vi "Move Absolute Motor.vi"(6 "Position":dbl min=-2000000000.0 max=2000000000.0 format="%.6f", 7 "timeout":dbl, 8 "error in (no error)":errorcluster, 9 "Axis":i32=1 min=1 max=3, 10 "VISA resource name in":refnum<visa-resource-name>, 11 "ESP302 in":refnum<class "ESP302.lvclass">) -> (0 "error out":errorcluster, 2 "VISA resource name out":refnum<visa-resource-name>, 3 "ESP302 out":refnum<class "ESP302.lvclass">)   [LabVIEW 2020, in "ESP302.lvclass"]
uses:
  ESP302.lvclass
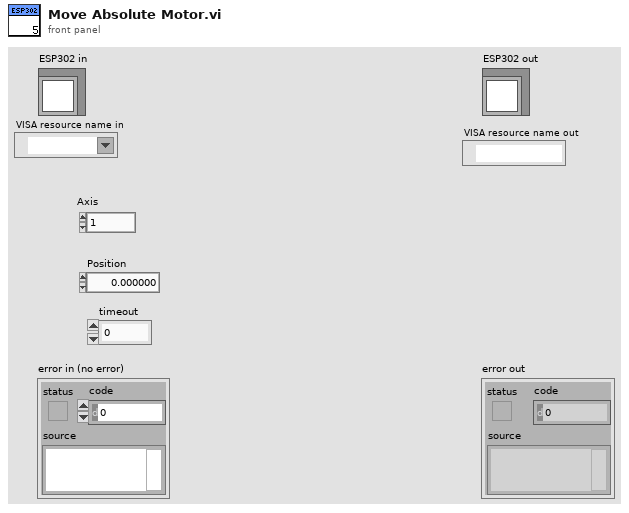
[diagram p1: front panel]
types:
  T1 = typedef "ESP301.lvclass/SettingsTypdef.ctl" = cluster{"devport":string, "Position":cluster{"Axis 1":cluster{"Value":dbl, "Min":dbl, "Max":dbl, "StepSize":dbl, "Tolerance":dbl, "ValueActual":dbl}, "Axis 2":cluster{"Value":dbl, "Min":dbl, "Max":dbl, "StepSize":dbl, "Tolerance":dbl, "ValueActual":dbl}, "Axis 3":cluster{"Value":dbl, "Min":dbl, "Max":dbl, "StepSize":dbl, "Tolerance":dbl, "ValueActual":dbl}}, "Power":cluster{"Axis 1":T2, "Axis 2":T2, "Axis 3":T2}, "Status":cluster{"Axis 1":T3, "Axis 2":T3, "Axis 3":T3}, "Backlash":cluster{"Axis 1":cluster{"Value":dbl, "Min":dbl, "Max":dbl, "StepSize":dbl, "Tolerance":dbl, "ValueActual":dbl}, "Axis 2":cluster{"Value":dbl, "Min":dbl, "Max":dbl, "StepSize":dbl, "Tolerance":dbl, "ValueActual":dbl}, "Axis 3":cluster{"Value":dbl, "Min":dbl, "Max":dbl, "StepSize":dbl, "Tolerance":dbl, "ValueActual":dbl}}, "Home":cluster{"Axis 1":cluster{"Value":dbl, "Min":dbl, "Max":dbl, "StepSize":dbl, "Tolerance":dbl, "ValueActual":dbl}, "Axis 2":cluster{"Value":dbl, "Min":dbl, "Max":dbl, "StepSize":dbl, "Tolerance":dbl, "ValueActual":dbl}, "Axis 3":cluster{"Value":dbl, "Min":dbl, "Max":dbl, "StepSize":dbl, "Tolerance":dbl, "ValueActual":dbl}}, "MoveToHardLimit":cluster{"Axis 1":T4, "Axis 2":T4, "Axis 3":T4}, "relativeMove":cluster{"Axis 1neg":T2, "Axis 2neg":T2, "Axis 3neg":T2, "Axis 1pos":T2, "Axis 2pos":T2, "Axis 3pos":T2}, "stepsize":cluster{"Value":dbl, "Min":dbl, "Max":dbl, "StepSize":dbl, "Tolerance":dbl, "ValueActual":dbl}, "automotoroff":T2, "ResetBeforeMove":T2, "Enable":cluster{"Axis 1":T2, "Axis 2":T2, "Axis 3":T2}, "InitWithDBValues":T2}
  T2 = typedef "OnOffTypeDef.ctl" = enum16{"off", "on"}
  T3 = typedef "status_TypDef.ctl" = enum16{"Not referenced", "Homing", "Moving", "Ready"}
  T4 = typedef "Hardware limit.ctl" = enum16{"pos", "neg"}
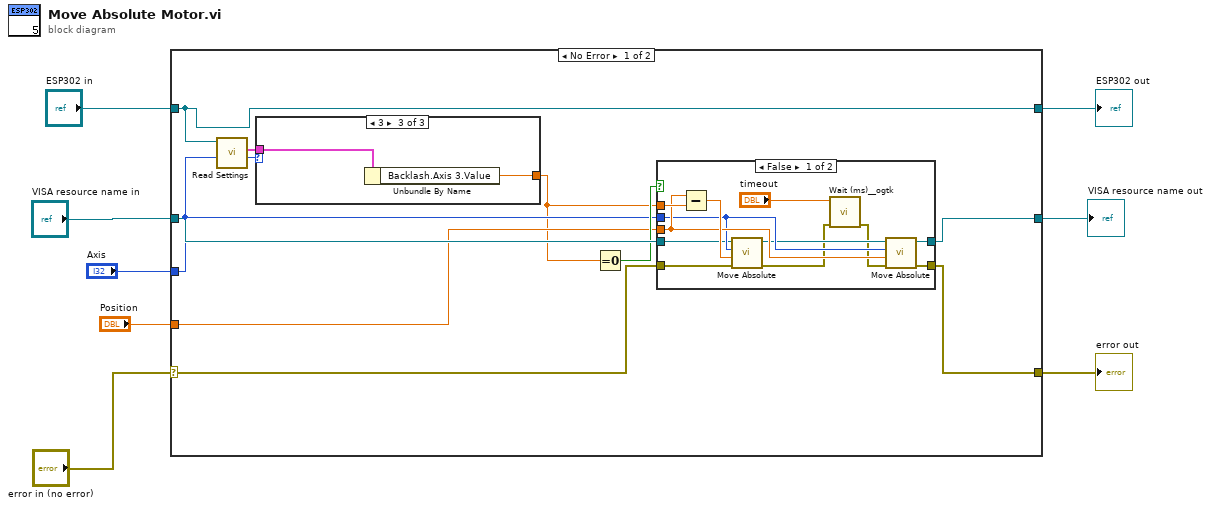
[diagram p0: block diagram]
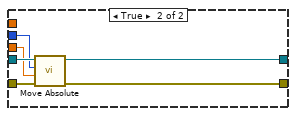
[diagram p2: hidden frame]
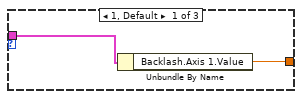
[diagram p3: hidden frame]
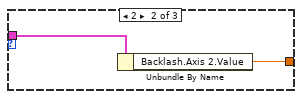
[diagram p4: hidden frame]
diagram:
  n1 = case shown="No Error" "error in (no error)" {
    selector: "error in (no error)" -> [w13 w45]
    tunnel: [w12 w45] -> w7
    tunnel: [w11 w44] -> w5
    tunnel: "ESP302 in" -> [w11 w44]
    tunnel: "VISA resource name in" -> [w18 w43]
    tunnel: [w17 w43] -> w3
    tunnel: "Axis" -> [w15 _]
    tunnel: "Position" -> [w14 _]
    frame No Error {
      n2 = call-dynamic "Read Settings.vi"("ESP301 in"=w11) -> ("Settings"=w10:T1)  [unwired: 8 in, 2 out]
      n3 = case shown="3" w15 {
        tunnel: w10 -> [w37 w40 w42]
        tunnel: [w38 w39 w41] -> w9
        frame 1, Default {
          n4 = Unbundle By Name(w37) -> ("Backlash.Axis 1.Value"=w38:dbl)
        }
        frame 2 {
          n5 = Unbundle By Name(w40) -> ("Backlash.Axis 2.Value"=w39:dbl)
        }
        frame 3 {
          n6 = Unbundle By Name(w42) -> ("Backlash.Axis 3.Value"=w41:dbl)
        }
      }
      n7 = Equal To 0?(x=w9) -> (x = 0?=w16:bool)
      n8 = case shown="False" w16 {
        tunnel: w18 -> [w24 w36]
        tunnel: [w23 w35] -> w17
        tunnel: w15 -> [w26 w34]
        tunnel: w14 -> [w27 w33]
        tunnel: w13 -> [w28 w32]
        tunnel: [w22 w31] -> w12
        tunnel: w9 -> [w30 _]
        frame False {
          n9 = Subtract(x=w27, y=w30) -> (x-y=w29:dbl)
          n10 = call "Move Absolute.vi"("error in (no error)"=w28, "Position (0 units)"=w29, "Axis (1)"=w26, "VISA resource name"=w24) -> ("error out"=w21:errorcluster, "VISA resource name out"=w25:refnum<visa-resource-name>)  [unwired: 2 in]
          n11 = call <userlib>:"Wait (ms)__ogtk.vi"("error in (no error)"=w21, "milliseconds to wait"="timeout") -> ("error out"=w20:errorcluster)  [unwired: 8 in, 1 out]
          n12 = call "Move Absolute.vi"("error in (no error)"=w20, "Position (0 units)"=w27, "Axis (1)"=w26, "VISA resource name"=w25) -> ("error out"=w22:errorcluster, "VISA resource name out"=w23:refnum<visa-resource-name>)  [unwired: 2 in]
        }
        frame True {
          n13 = call "Move Absolute.vi"("error in (no error)"=w32, "Position (0 units)"=w33, "Axis (1)"=w34, "VISA resource name"=w36) -> ("error out"=w31:errorcluster, "VISA resource name out"=w35:refnum<visa-resource-name>)  [unwired: 2 in]
        }
      }
    }
    frame Error {
    }
  }
  "error out" <- w7
  "ESP302 out" <- w5
  "VISA resource name out" <- w3
